vi "Examne.vi"() -> ()   [LabVIEW 2020]
uses:
  <vilib>/numeric/Random Number (Range) U64.vi
  <vilib>/numeric/sub_Random U32.vi
panel:
  out "Numeros  que pasan el maximo":i16
  in  "stop":bool
  out "Waveform Chart":cluster{"number":u64, dbl}[](graph)
  out "Numero":u64
  out "Histeresis":bool
  out "Rango":bool
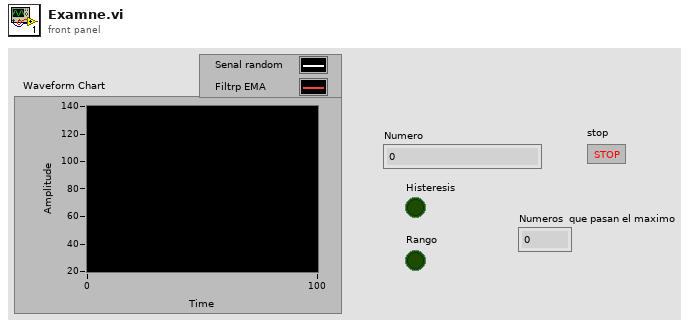
[diagram p1: front panel]
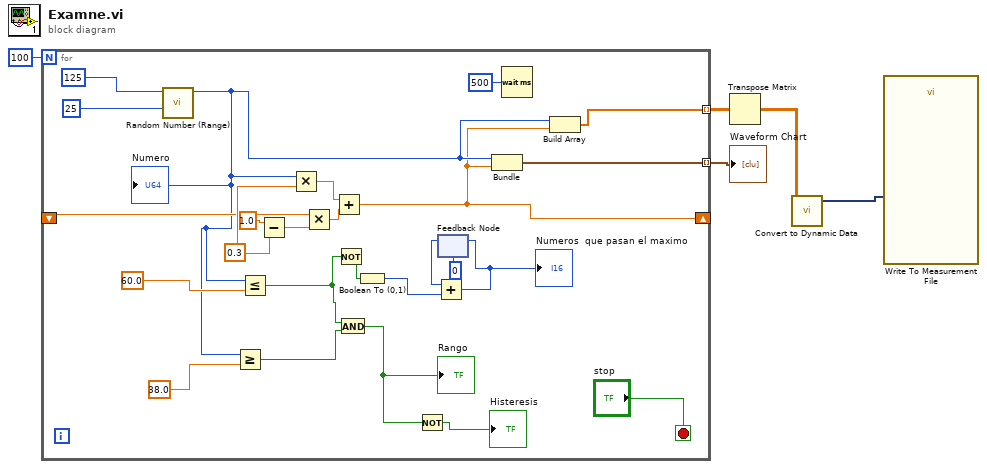
[diagram p0: block diagram]
diagram:
  n1 = for {
    N: 100 -> [_]
    shift-right: [w7] -> _
    shift-left: _ -> [w17]
    tunnel: [w16] -> w5 mode=indexing
    tunnel: [w6] -> w3 mode=indexing
    stop <- "stop" stop-if-true
    w18 = 0.3 ("y")
    n2 = call-poly <vilib>:"Random Number (Range).vi"("lower bound (0)"=u64 25, "upper bound (100)"=u64 125) -> ("number"=w8:u64)  [unwired: 9 in]
    "Numero" <- w8
    n3 = Greater Or Equal?(x=w8, y=38.0 ("Min")) -> (x >= y?=w25:bool)
    n4 = Less Or Equal?(x=w8, y=60.0 ("Max")) -> (x <= y?=w14:bool)
    n5 = Subtract(x=1.0, y=w18) -> (x-y=w20:dbl)
    n6 = Multiply(x=w8, y=w18) -> (x*y=w22:dbl)
    n7 = Multiply(x=w17, y=w20) -> (x*y=w21:dbl)
    n8 = Add(x=w22, y=w21) -> (x+y=w7:dbl)
    n9 = Not(x=w14) -> (.not. x?=w13:bool)
    n10 = And(x=w14, y=w25) -> (x .and. y?=w24:bool)
    "Rango" <- w24
    n11 = Boolean To (0,1)(Boolean=w13) -> (0, 1=w15:i16)
    n12 = Not(x=w24) -> (.not. x?=→"Histeresis":bool)
    n13 = feedback #1(i16 0) -> (w12:i16)
    n14 = Add(x=w12, y=w15) -> (x+y=w11:i16)
    "Numeros  que pasan el maximo" <- w11
    n15 = feedback-in #1(w11) -> ()
    n16 = Bundle("number"=w8, w7) -> (w16:cluster{"number":u64, dbl})  [unwired: 1 in]
    n17 = Wait (ms)(milliseconds to wait=u32 500) -> ()  [unwired: 1 out]
    n18 = Build Array "Build Array"(w8, w7) -> (w6:dbl[])
  }
  "Waveform Chart" <- w5
  n19 = Transpose Matrix(1:w3) -> (0:w2:dbl[][])
  n20 = call "Convert to Dynamic Data"("2D Array"=w2) -> ("Dynamic Data Type"=w1:dynamicdata)  [unwired: 3 in]
  n21 = call "Write To Measurement File"("Signals"=w1) -> ()  [unwired: 16 in, 3 out]
